vi "Receiver.vi"() -> ()   [LabVIEW 2013]
uses:
  <vilib>/sound2/lvsound2.llb/Sound Data Format.ctl
  <instrlib>/niUSRP/niUSRP Fetch Rx Data (CDB WDT).vi
  <vilib>/Analysis/2dsp.llb/Rational Resample (single channel, DBL).vi
  <vilib>/sound2/lvsound2.llb/Sound Output Write (DBL Single).vi
  <vilib>/express/express analysis/Spectral/Block/exnSpectralBlock spectral measurements RMS poly.vi
  <vilib>/express/express analysis/Spectral/Block/exnSpectralBlock spectral measurements RMS WFM.vi
  <vilib>/express/express analysis/Spectral/XNode/ExpressSpectralMeasurementsBlockNode.xnode
  <vilib>/Analysis/NI_AALPro.lvlib
panel:
  in  "stop":bool
  out "Spectrum(FFT)":cluster{"f0":dbl, "df":dbl, "magnitude":dbl[]}(graph)
  in  "device names":refnum<k15>="192.168.10.2"
  out "XY Graph":cluster{dbl[], dbl[]}(graph)
  out "error out 2":errorcluster
  out "error out":errorcluster
  in  "sound format":T1={"sample rate (S/s)"=44100.0, "number of channels"=1, "bits per sample"=16}
  in  "number of samples":i32=44100
  in  "active antenna":string="RX2"
  out "coerced gain":dbl format="%#_6p"
  out "coerced carrier frequency":dbl=100000.0 format="%#_6p"
  out "coerced IQ rate":dbl=200000.0 format="%#_6p"
  in  "gain":dbl(knob) scale=0.0..10.0
  in  "carrier frequency":dbl=2400000000.0 format="%#_6p"
  in  "IQ rate":dbl=200000.0 format="%#_6p"
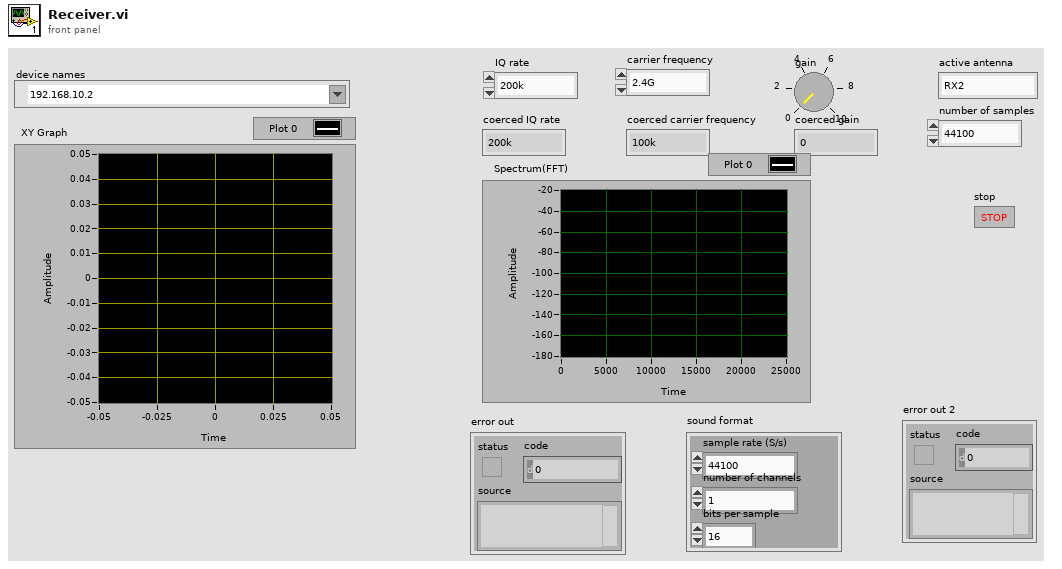
[diagram p1: front panel]
types:
  T1 = typedef "Sound Data Format.ctl" = cluster{"sample rate (S/s)":dbl, "number of channels":i32, "bits per sample":i32}
  T2 = typedef "Sound Output Task ID.ctl" = u32
  T3 = cluster{"averaging mode":u16, "weighting mode":u16, "number of averages":u32}
  T4 = cluster{"dB On (F)":bool, "unwrap phase (F)":bool, "convert to degree (F)":bool}
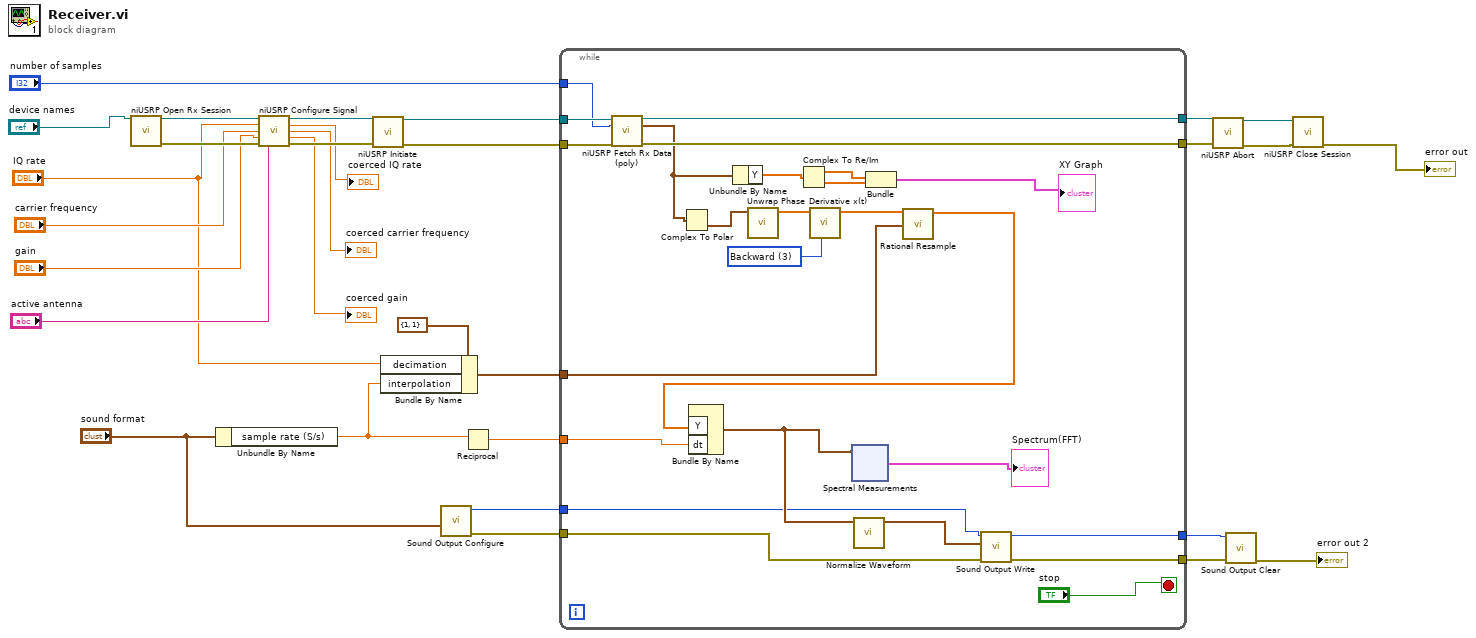
[diagram p0: block diagram]
diagram:
  n1 = call <instrlib>:"niUSRP Open Rx Session.vi"("device names"="device names") -> ("session handle out"=w30:refnum<k15>, "error out"=w29:errorcluster)  [unwired: 13 in]
  n2 = Unbundle By Name("sound format") -> ("sample rate (S/s)"=w20:dbl)
  n3 = call <instrlib>:"niUSRP Configure Signal.vi"("session handle"=w30, "IQ rate"="IQ rate", "carrier frequency"="carrier frequency", "gain"="gain", "error in (no error)"=w29, "active antenna"="active antenna") -> ("session handle out"=w24:refnum<k15>, "coerced IQ rate"=→"coerced IQ rate":dbl, "coerced carrier frequency"=→"coerced carrier frequency":dbl, "coerced gain"=→"coerced gain":dbl, "error out"=w25:errorcluster)  [unwired: 5 in]
  n4 = call <instrlib>:"niUSRP Initiate.vi"("session handle"=w24, "error in (no error)"=w25) -> ("session handle out"=w17:refnum<k15>, "error out"=w16:errorcluster)  [unwired: 12 in]
  n5 = Bundle By Name(cluster=cluster{"interpolation":i32, "decimation":i32} {"interpolation"=1, "decimation"=1} ("input cluster"), "decimation"="IQ rate", "interpolation"=w20) -> (w9:cluster{"interpolation":i32, "decimation":i32})
  n6 = call <vilib>:"Sound Output Configure.vi"("sound format"="sound format") -> ("error out"=w6:errorcluster, "task ID"=w7:T2)  [unwired: 9 in]
  n7 = Reciprocal(x=w20) -> (1/x=w8:dbl)
  n8 = while {
    tunnel: w17 -> [w55]
    tunnel: w16 -> [w54]
    tunnel: "number of samples" -> [w53]
    tunnel: [w52] -> w14
    tunnel: [w51] -> w12
    tunnel: w9 -> [w43]
    tunnel: w8 -> [w40]
    tunnel: w7 -> [w37]
    tunnel: w6 -> [w36]
    tunnel: [w35] -> w4
    tunnel: [w34] -> w3
    stop <- "stop" stop-if-true
    w42 = u16 3 items=["2nd Order Central", "4th Order Central", "Forward", "Backward"] ("method")
    n9 = call-poly <instrlib>:"niUSRP Fetch Rx Data (poly).vi"("session handle"=w55, "number of samples"=w53, "error in (no error)"=w54) -> ("session handle out"=w52:refnum<k15>, "data"=w50:waveform(cdb), "error out"=w51:errorcluster)  [unwired: 9 in, 1 out]
    n10 = Complex To Polar(r * e^(i*theta)=w50) -> (theta=w48:waveform(dbl))  [unwired: 1 out]
    n11 = Unbundle By Name(w50) -> ("Y"=w49:cdb[])
    n12 = call <vilib>:"Unwrap Phase.vi"("Phase"=w48) -> ("Unwrapped Phase"=w45:dbl[])  [unwired: 9 in, 1 out]
    n13 = Complex To Re/Im(x + iy=w49) -> (x=w47:dbl[], y=w46:dbl[])
    n14 = call <vilib>:"Derivative x(t).vi"("method"=w42, "X"=w45) -> ("dX/dt"=w44:dbl[])  [unwired: 8 in, 1 out]
    n15 = Bundle(w47, w46) -> (→"XY Graph":cluster{dbl[], dbl[]})  [unwired: 1 in]
    n16 = call-poly <vilib>:"Rational Resample.vi"("resample factor"=w43, "X"=w44) -> ("Y"=w41:dbl[])  [unwired: 7 in, 2 out]
    n17 = Bundle By Name("Y"=w41, "dt"=w40) -> (w38:waveform(dbl))  [unwired: 1 in]
    n18 = xnode "Spectral Measurements"("Signals"=w38) -> ("FFT - (RMS)"=→"Spectrum(FFT)":cluster{"f0":dbl, "df":dbl, "magnitude":dbl[]})  [unwired: 1 in, 2 out]
    n19 = call <vilib>:"Normalize Waveform.vi"("waveform in"=w38) -> ("normalized waveform"=w39:waveform(dbl))  [unwired: 7 in, 3 out]
    n20 = call-poly <vilib>:"Sound Output Write.vi"("error in (no error)"=w36, "data"=w39, "task ID"=w37) -> ("error out"=w34:errorcluster, "task ID out"=w35:T2)  [unwired: 7 in]
  }
  n21 = call <instrlib>:"niUSRP Abort.vi"("session handle"=w14, "error in (no error)"=w12) -> ("session handle out"=w13:refnum<k15>, "error out"=w11:errorcluster)  [unwired: 12 in]
  n22 = call <vilib>:"Sound Output Clear.vi"("error in (no error)"=w3, "task ID"=w4) -> ("error out"=→"error out 2":errorcluster)  [unwired: 9 in]
  n23 = call <instrlib>:"niUSRP Close Session.vi"("session handle"=w13, "error in (no error)"=w11) -> ("error out"=→"error out":errorcluster)  [unwired: 13 in]
